vi "SigProc_subVI scriptAnalyser.vi"(1 "Script in":string) -> (0 "Variables out":T1(array[cluster]))   [LabVIEW 2018, in "Sig2MS.lvclass"]
uses:
  Sig2MS.lvclass
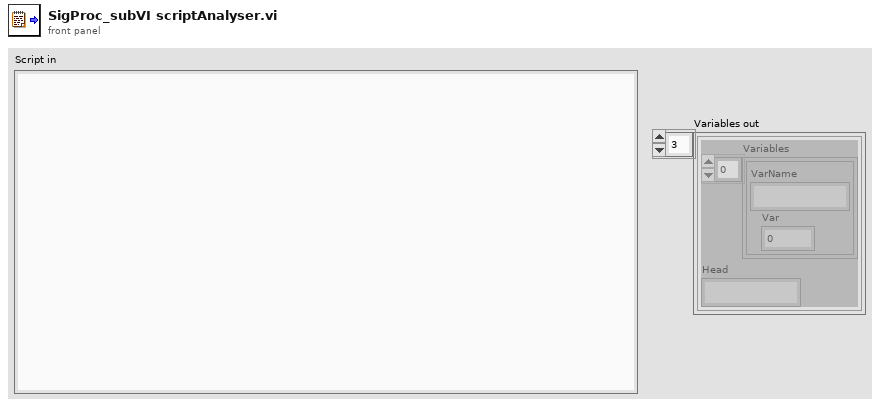
[diagram p1: front panel]
types:
  T1 = cluster{"Variables":cluster{"VarName":string, "Var":dbl}[], "Head":string}[]
  T2 = cluster{"Variables":cluster{"VarName":string, "Var":dbl}[], "Head":string}
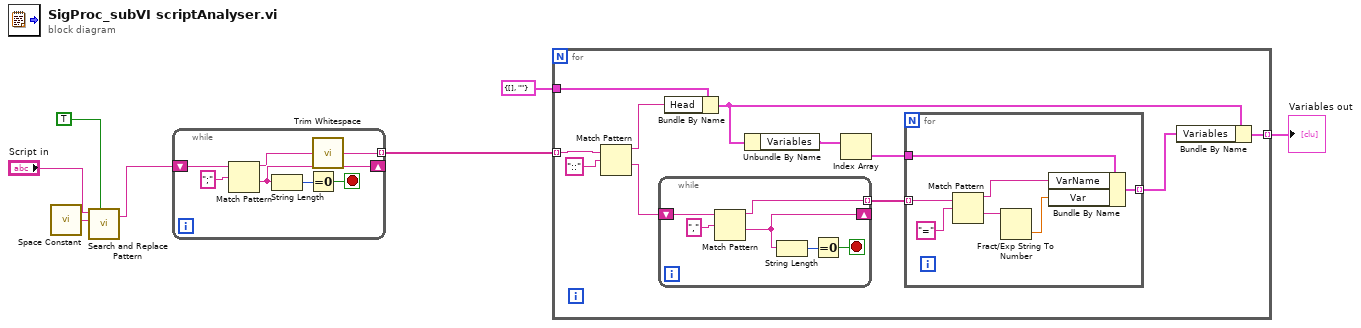
[diagram p0: block diagram]
diagram:
  n1 = call <vilib>:"Space Constant.vi"() -> ("String"=w3:string)
  n2 = call <vilib>:"Search and Replace Pattern.vi"("string"="Script in", "regular expression (\"\")"=w3, "replace all? (F)"=TRUE) -> ("result string"=w1:string)  [unwired: 2 in, 1 out]
  n3 = while {
    shift-right: [w12] -> _
    shift-left: w1 -> [w14]
    tunnel: [w8] -> w7 mode=indexing
    stop <- w10 stop-if-true
    n4 = Match Pattern(string=w14, regular expression=";") -> (before substring=w9:string, after substring=w12:string)  [unwired: 1 in, 2 out]
    n5 = String Length(string=w12) -> (length=w11:i32)
    n6 = Equal To 0?(x=w11) -> (x = 0?=w10:bool)
    n7 = call <vilib>:"Trim Whitespace.vi"("string"=w9) -> ("trimmed string"=w8:string)  [unwired: 1 in]
  }
  n8 = for {
    tunnel: w7 -> [w25] mode=indexing
    tunnel: T2 {"Variables"=[], "Head"=""} -> [w23]
    tunnel: [w15] -> w5 mode=indexing
    n9 = Match Pattern(string=w25, regular expression="::") -> (before substring=w22:string, after substring=w21:string)  [unwired: 1 in, 2 out]
    n10 = while {
      shift-right: [w35] -> _
      shift-left: w21 -> [w38]
      tunnel: [w36] -> w20 mode=indexing
      stop <- w33 stop-if-true
      n11 = Match Pattern(string=w38, regular expression=",") -> (before substring=w36:string, after substring=w35:string)  [unwired: 1 in, 2 out]
      n12 = String Length(string=w35) -> (length=w34:i32)
      n13 = Equal To 0?(x=w34) -> (x = 0?=w33:bool)
    }
    n14 = Bundle By Name(cluster=w23, "Head"=w22) -> (w16:T2)
    n15 = Unbundle By Name(w16) -> ("Variables"=w19:cluster{"VarName":string, "Var":dbl}[])
    n16 = Index Array(array=w19) -> (element=w18:cluster{"VarName":string, "Var":dbl})  [unwired: 1 in]
    n17 = for {
      tunnel: w20 -> [w32] mode=indexing
      tunnel: w18 -> [w30]
      tunnel: [w26] -> w17 mode=indexing
      n18 = Match Pattern(string=w32, regular expression="=") -> (before substring=w29:string, after substring=w28:string)  [unwired: 1 in, 2 out]
      n19 = Fract/Exp String To Number(string=w28) -> (number=w27:dbl)  [unwired: 3 in, 1 out]
      n20 = Bundle By Name(cluster=w30, "VarName"=w29, "Var"=w27) -> (w26:cluster{"VarName":string, "Var":dbl})
    }
    n21 = Bundle By Name(cluster=w16, "Variables"=w17) -> (w15:T2)
  }
  "Variables out" <- w5
